vi "Get Variable Channel Linkages.vi"(8 "error in (no error)":errorcluster, 10 "Linked Channels":T1[](array[typedef]), 11 "Item Ref in":T2 format="%.0x") -> (0 "error out":errorcluster, 2 "Array":string[][](array[string]), 3 "Item Ref out":T2 format="%.0x")   [LabVIEW 2018, in "Instrument Addon System Explorer.lvlib"]
uses:
  Instrument Addon System Explorer.lvlib
  <vilib>/NI Veristand/Custom Device API/Custom Device Item Ref.ctl
  Addon Shared/Types/Linked Channel Cluster.ctl
  NationalInstruments.VeriStand.SystemStorage
  Addon Shared/SubVIs/Constants.vi
  <vilib>/NI Veristand/Custom Device Tools/Custom Device Utility Library/NI VeriStand - Search for Item by Property.vi
  <vilib>/NI VeriStand/Custom Device API/Custom Device API.lvlib
  <vilib>/NI VeriStand/Custom Device Tools/Custom Device Utility Library/Custom Device Utility Library.lvlib
  Addon Shared/Instrument Addon Shared.lvlib
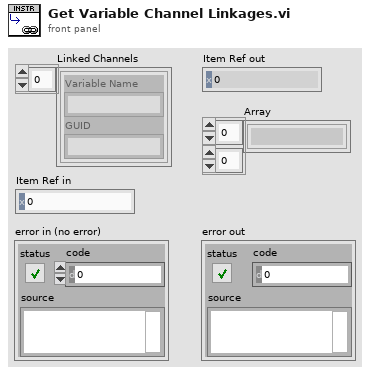
[diagram p1: front panel]
types:
  T1 = typedef "Instrument Addon Shared.lvlib/Linked Channel Cluster.ctl" = cluster{"Variable Name":string, "GUID":string}
  T2 = typedef "Custom Device API.lvlib/Custom Device Item Ref.ctl" = u64
  T3 = typedef "Custom Device API.lvlib/Custom Device Pointer.ctl" = refnum<k24>
  T4 = typedef "Custom Device API.lvlib/Custom Device Item Info.ctl" = cluster{"Name":string, "Is Channel":bool, "GUID":string, "Is Waveform":bool}
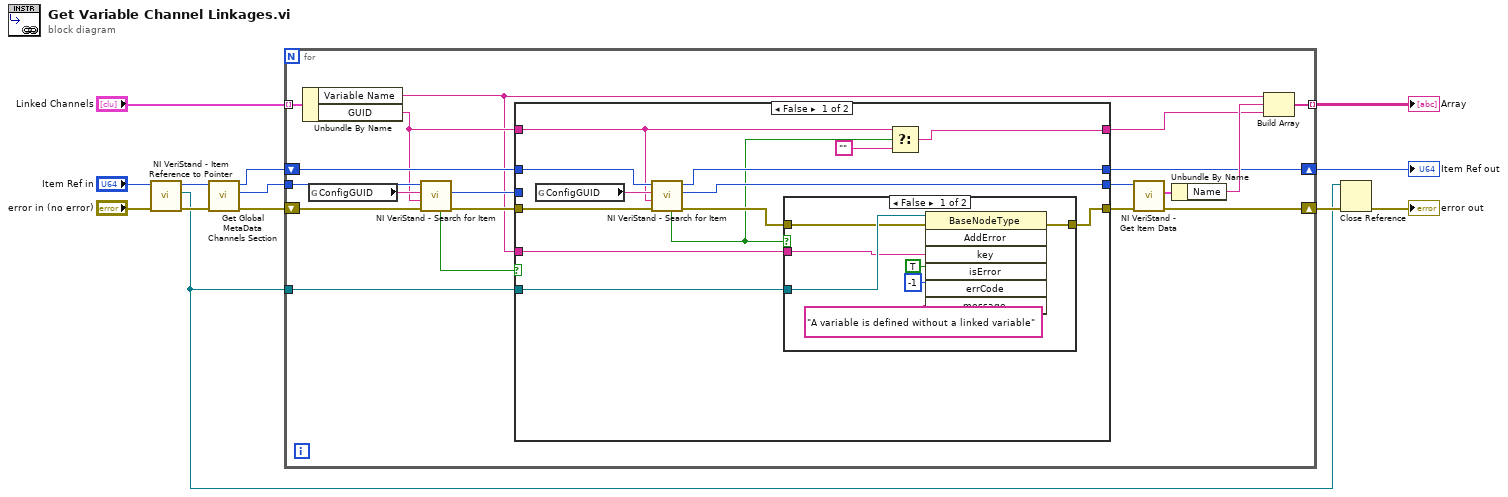
[diagram p0: block diagram]
diagram:
  n1 = call <vilib>:"NI VeriStand - Item Reference to Pointer.vi"("error in (no error)"="error in (no error)", "Item Ref in"="Item Ref in") -> ("error out"=w3:errorcluster, "Node Pointer"=w1:T3, "Item Ref out"=w5:T2)  [unwired: 6 in, 1 out]
  n2 = call "Get Global MetaData Channels Section.vi"("error in (no error)"=w3, "Item Ref in"=w5) -> ("error out"=w11:errorcluster, "Item Ref"=w8:T2, "Item Ref out"=w9:T2)  [unwired: 7 in]
  n3 = for {
    tunnel: "Linked Channels" -> [w31] mode=indexing
    shift-right: [w30] -> w6
    shift-left: w11 -> [w27]
    tunnel: [w28] -> w12 mode=indexing
    tunnel: w8 -> [w26]
    shift-right: [w17] -> w10
    shift-left: w9 -> [w19]
    tunnel: w1 -> [w15]
    n4 = Unbundle By Name(w31) -> ("Variable Name"=w14:string, "GUID"=w18:string)
    n5 = global read "Constants.vi" "ConfigGUID"() -> (w25:string)
    n6 = call-poly <vilib>:"NI VeriStand - Search for Item.vi"("error in"=w27, "Property Value"=w18, "Property Name"=w25, "Section Ref in"=w26) -> ("error out"=w22:errorcluster, "Item Ref"=w20:T2, "Found"=w24:bool)  [unwired: 4 in, 1 out]
    n7 = case shown="False" w24 {
      tunnel: [w35 w57] -> w23
      tunnel: w22 -> [w45 w57]
      tunnel: [w44 w56] -> w21
      tunnel: w20 -> [_ w56]
      tunnel: w19 -> [w43 w55]
      tunnel: w18 -> [w40 w54]
      tunnel: [w41 w55] -> w17
      tunnel: [w38 w54] -> w16
      tunnel: w15 -> [w37 _]
      tunnel: w14 -> [w34 _]
      frame False {
        n8 = global read "Constants.vi" "ConfigGUID"() -> (w42:string)
        n9 = call-poly <vilib>:"NI VeriStand - Search for Item.vi"("error in"=w45, "Property Value"=w40, "Property Name"=w42, "Section Ref in"=w43) -> ("error out"=w36:errorcluster, "Item Ref"=w44:T2, "Section Ref out"=w41:T2, "Found"=w33:bool)  [unwired: 4 in]
        n10 = case shown="False" w33 {
          tunnel: w37 -> [w52 _]
          tunnel: w36 -> [w51 w53]
          tunnel: [w50 w53] -> w35
          tunnel: w34 -> [w49 _]
          frame False {
            n11 = invoke class="BaseNodeType" method="AddError"(reference=w52, error in=w51, "key"=w49, "isError"=TRUE, "errCode"=-1, "message"="A variable is defined without a linked variable") -> (error out=w50:errorcluster)  [unwired: 1 in, 6 out]
          }
          frame True {
          }
        }
        n12 = Select(t=w40, s=w33, f="") -> (s? t:f=w38:string)
      }
      frame True {
      }
    }
    n13 = call <vilib>:"NI VeriStand - Get Item Data.vi"("error in (no error)"=w23, "Item Ref in"=w21) -> ("error out"=w30:errorcluster, "Item Info"=w32:T4)  [unwired: 8 out]
    n14 = Unbundle By Name(w32) -> ("Name"=w29:string)
    n15 = Build Array(w14, w29, w16) -> (w28:string[])
  }
  "Array" <- w12
  "Item Ref out" <- w10
  n16 = Close Reference(reference=w1, error in (no error)=w6) -> (error out=→"error out":errorcluster)
